vi "Read Element of V.vi"(8 "error in (no error)":errorcluster, 10 "index":i32, 11 "IV_data in":refnum<class "IV_data.lvclass">) -> (0 "error out":errorcluster, 2 "Numeric":dbl, 3 "IV_data out":refnum<class "IV_data.lvclass">)   [LabVIEW 2014, in "IV_data.lvclass"]
uses:
  IV_data.lvclass
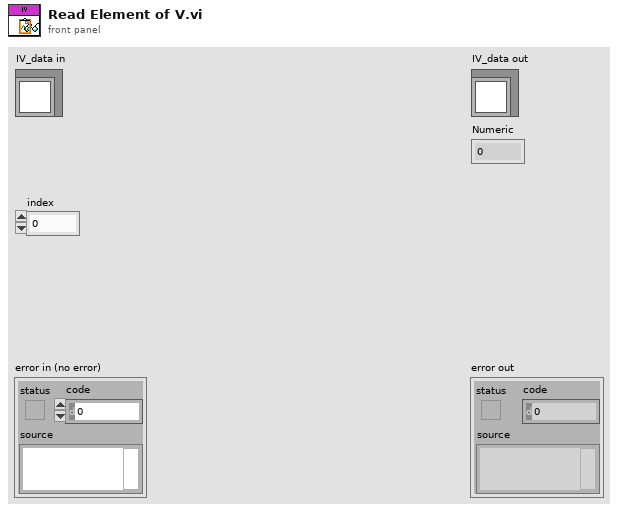
[diagram p1: front panel]
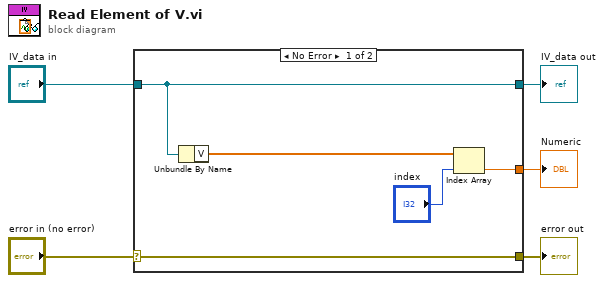
[diagram p0: block diagram]
diagram:
  n1 = case shown="No Error" "error in (no error)" {
    selector: "error in (no error)" -> [w10 w11]
    tunnel: [w10 w11] -> w4
    tunnel: [w9 w12] -> w2
    tunnel: "IV_data in" -> [w9 w12]
    tunnel: [w6 _] -> w1
    frame No Error {
      n2 = Unbundle By Name(w9) -> ("V"=w8:dbl[])
      n3 = Index Array(array=w8, index="index") -> (element=w6:dbl)
    }
    frame Error {
    }
  }
  "error out" <- w4
  "IV_data out" <- w2
  "Numeric" <- w1
